vi "upload.complete_multipart_upload.vi"(8 "error in":errorcluster, 11 "Multipart Upload in":refnum<class "Multipart Upload.lvclass">) -> (0 "error out":errorcluster, 2 "S3 Path to File":string)   [LabVIEW 2020, in "Multipart Upload.lvclass"]
doc: "Completes a multipart upload to S3. This should be called after all parts have been uploaded."
uses:
  Nominal Client MultiPart Upload/Multipart Upload.lvclass
  Nominal Client MultiPart Upload/Multipart Upload.lvclass/Multipart Upload.ctl
  8b3dcdab-c30a-41f7-882b-0fd92512159b.vi
  Nominal Client MultiPart Upload/nominal_client.get.vi
  Nominal Client MultiPart Upload/parts.get.vi
  <vilib>/JDP Science/JSONtext/JSON text to Variant.vi
  Nominal Client.lvclass
  <vilib>/JDP Science/JSONtext/LVClass Serializer/JSONtext LVClass Serializer.lvclass
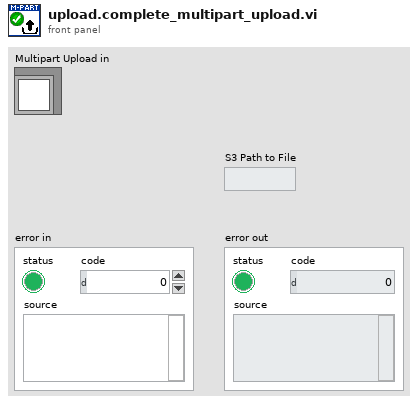
[diagram p1: front panel]
types:
  T1 = cluster{"partNumber":i32, "etag":string, "size":i32}[]
  T2 = cluster{"Part Number":i32, "ETag":string, "Size":i32}[]
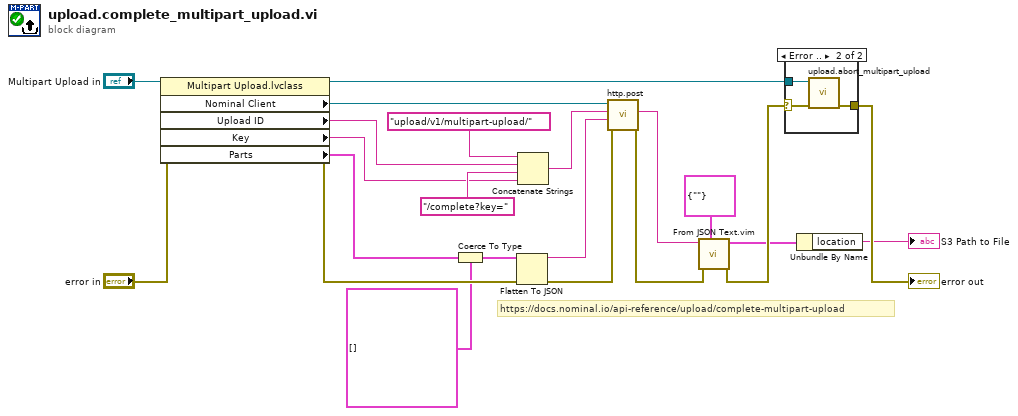
[diagram p0: block diagram]
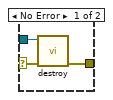
[diagram p2: hidden frame]
diagram:
  # "https://docs.nominal.io/api-reference/upload/complete-multipart-upload"
  n1 = property class="Multipart Upload.lvclass"(reference="Multipart Upload in", error in="error in") -> (reference out=w8:refnum<class "Multipart Upload.lvclass">, error out=w12:errorcluster, "Nominal Client"=w9:refnum<class "Nominal Client.lvclass">, "Upload ID"=w14:string, "Key"=w13:string, "Parts"=w4:T2)
  n2 = Coerce To Type(0:w4, 1:T1 [] ("anything")) -> (2:w3:T1)
  n3 = Flatten To JSON(anything=w3, error in (no error)=w12) -> (JSON string=w16:string, 11:w17:errorcluster)  [unwired: 1 in]
  n4 = Concatenate Strings("upload/v1/multipart-upload/" ("Path"), w14, "/complete?key=" ("string"), w13) -> (w19:string)
  n5 = call "http.post.vi"("error in"=w17, "Request body"=w16, "Path"=w19, "Nominal Client in"=w9) -> ("error out"=w10:errorcluster, "Response"=w21:string)  [unwired: 4 in, 2 out]
  n6 = call "From JSON Text.vim"("Data Type and Default Value"=cluster{"location":string} {"location"=""}, "error in (no error)"=w10, "JSON"=w21) -> ("error out"=w7:errorcluster, "Data out"=w5:cluster{"location":string})  [unwired: 7 in]
  n7 = case shown="Error .." w7 {
    selector: w7 -> [w24 w27]
    tunnel: w8 -> [w25 w28]
    tunnel: [w23 w26] -> w6
    frame No Error {
      n8 = call "destroy.vi"("error in"=w24, "MultiPart Upload"=w25) -> ("error out"=w23:errorcluster)  [unwired: 9 in]
    }
    frame Error {
      n9 = call "upload.abort_multipart_upload.vi"("error in"=w27, "Multipart Upload"=w28) -> ("error out"=w26:errorcluster)  [unwired: 9 in]
    }
  }
  "error out" <- w6
  n10 = Unbundle By Name(w5) -> ("location"=→"S3 Path to File":string)
